vi "Configuracao.Leitura.vi"(8 "error in":errorcluster) -> (0 "error out":errorcluster)   [LabVIEW 2019]
uses:
  <vilib>/Utility/xml.llb/Read From XML File(string).vi
  Configuracao.Variaveis.vi
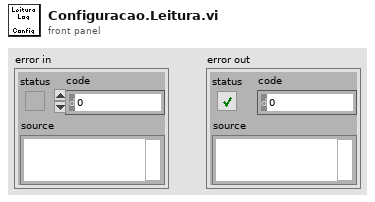
[diagram p1: front panel]
types:
  T1 = cluster{"TipoMedicao":string, "Medir":bool, "Medicao":dbl}
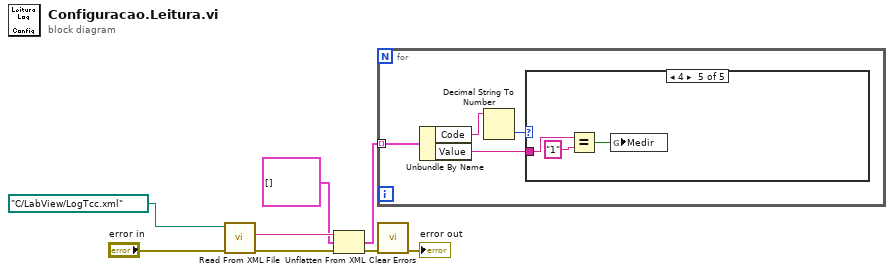
[diagram p0: block diagram]
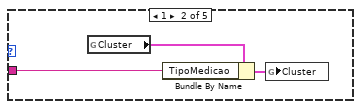
[diagram p3: hidden frame]
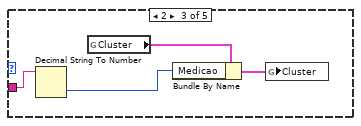
[diagram p4: hidden frame]
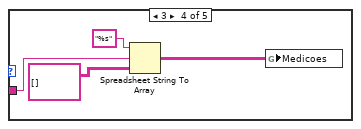
[diagram p5: hidden frame]
diagram:
  n1 = call-poly <vilib>:"Read From XML File.vi"("error in (no error)"="error in", "XML File Path"=path "C:/LabView/LogTcc.xml") -> ("error out"=w4:errorcluster, "XML Elements"=w8:string)  [unwired: 7 in, 1 out]
  n2 = Unflatten From XML(xml string=w8, type=cluster{"Code":string, "Value":string}[] [] ("anything"), error in (no error)=w4) -> (value=w6:cluster{"Code":string, "Value":string}[], error out=w3:errorcluster)
  n3 = for {
    tunnel: w6 -> [w12] mode=indexing
    n4 = Unbundle By Name(w12) -> ("Code"=w11:string, "Value"=w9:string)
    n5 = Decimal String To Number(string=w11) -> (number=w10:i32)  [unwired: 2 in, 1 out]
    n6 = case shown="4" w10 {
      tunnel: w9 -> [_ w13 w17 w21 w25]
      frame 0, Default {
      }
      frame 1 {
        n7 = global read "Configuracao.Variaveis.vi" "Cluster"() -> (w14:T1)
        n8 = Bundle By Name(cluster=w14, "TipoMedicao"=w13) -> (w15:T1)
        n9 = global write "Configuracao.Variaveis.vi" "Cluster"(w15) -> ()
      }
      frame 2 {
        n10 = Decimal String To Number(string=w17) -> (number=w16:i32)  [unwired: 2 in, 1 out]
        n11 = global read "Configuracao.Variaveis.vi" "Cluster"() -> (w18:T1)
        n12 = Bundle By Name(cluster=w18, "Medicao"=w16) -> (w19:T1)
        n13 = global write "Configuracao.Variaveis.vi" "Cluster"(w19) -> ()
      }
      frame 3 {
        n14 = Spreadsheet String To Array(format string="%s", spreadsheet string=w21, array type (2D Dbl)=string[][] []) -> (array=w20:string[][])  [unwired: 1 in]
        n15 = global write "Configuracao.Variaveis.vi" "Medicoes"(w20) -> ()
      }
      frame 4 {
        n16 = Equal?(x=w25, y="1") -> (x = y?=w24:bool)
        n17 = global write "Configuracao.Variaveis.vi" "Medir"(w24) -> ()
      }
    }
  }
  n18 = call <vilib>:"Clear Errors.vi"("error in (no error)"=w3) -> ("error out"=→"error out":errorcluster)  [unwired: 5 in, 1 out]
